vi "HeatFlow Stop Acq Tasks.vi"(9 "HeatFlow HW Cfg":T1, 11 "HeatFlow HW Tasks in":T2) -> (0 "error out":errorcluster)   [LabVIEW 2019, in "Acquisition.lvlib"]
doc: "Perform the acquisition. Replace the contents of this diagram with calls to acquisition hardware."
uses:
  Acquisition.lvlib
  HeatFlow HW Tasks.ctl
  HeatFlow HW Cfg.ctl
  HeatFlow Acq States.ctl
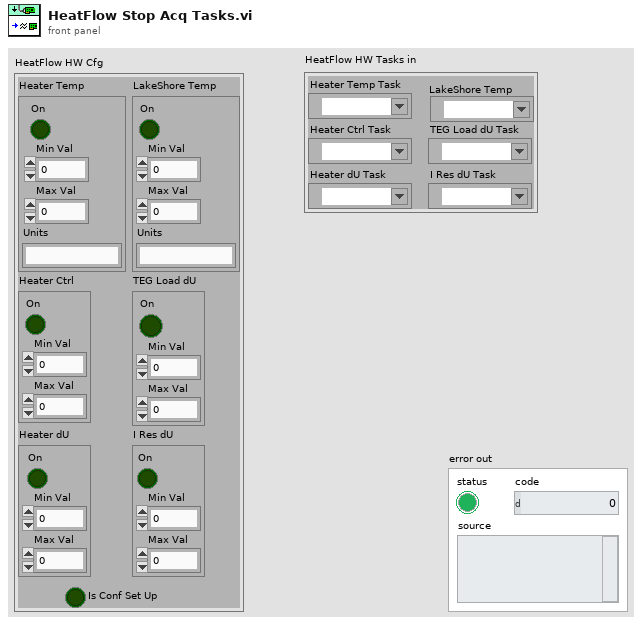
[diagram p1: front panel]
types:
  T1 = typedef "Acquisition.lvlib/HeatFlow HW Cfg.ctl" = cluster{"Heater Temp":cluster{"On":bool, "Min Val":dbl, "Max Val":dbl, "Units":string}, "LakeShore Temp":cluster{"On":bool, "Min Val":dbl, "Max Val":dbl, "Units":string}, "Heater Ctrl":cluster{"On":bool, "Min Val":dbl, "Max Val":dbl}, "TEG Load dU":cluster{"On":bool, "Min Val":dbl, "Max Val":dbl}, "Heater dU":cluster{"On":bool, "Min Val":dbl, "Max Val":dbl}, "I Res dU":cluster{"On":bool, "Min Val":dbl, "Max Val":dbl}, "Is Conf Set Up":bool}
  T2 = typedef "Acquisition.lvlib/HeatFlow HW Tasks.ctl" = cluster{"Heater Temp Task":refnum<k21>, "Heater Ctrl Task":refnum<k21>, "TEG Load dU Task":refnum<k21>, "Heater dU Task":refnum<k21>, "I Res dU Task":refnum<k21>, "LakeShore Temp":refnum<visa-resource-name>}
  T3 = typedef "Acquisition.lvlib/HeatFlow Acq States.ctl" = enum16{"Start", "--- Control ---", "HeaterTemp", "DoControl?", "HeaterCtrl", "--- Readings ---", "DoReadings?", "I_Res_dU", "LakeShoreTemp", "Heater_dU", "TEG_Load_dU", "Calculations", "End"}
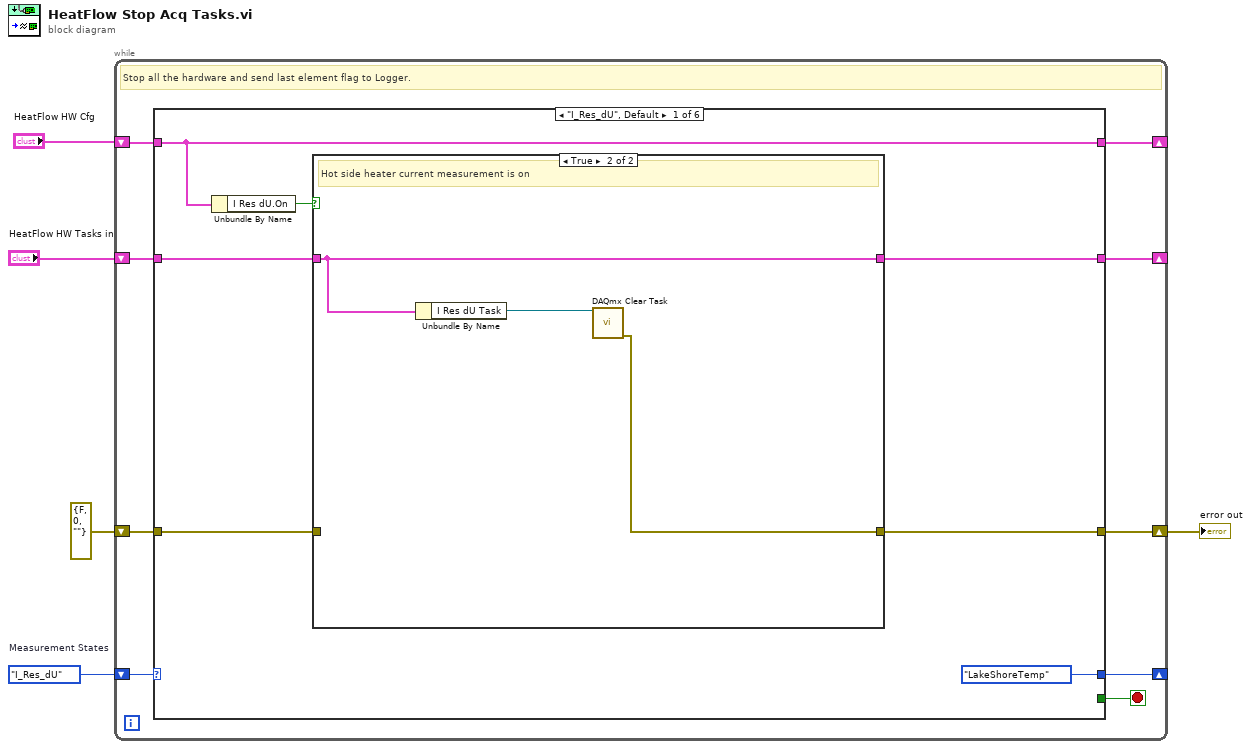
[diagram p0: block diagram]
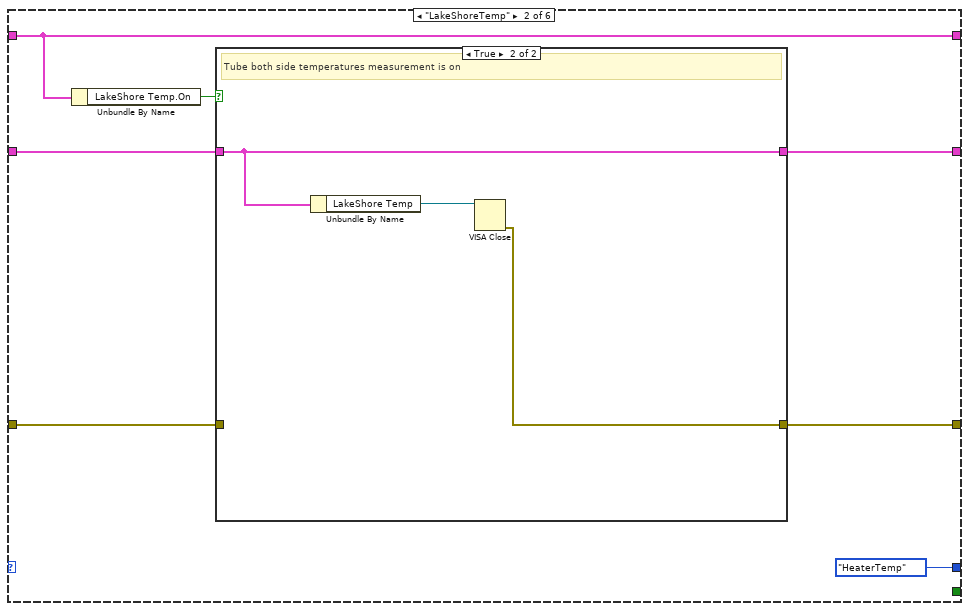
[diagram p3: hidden frame]
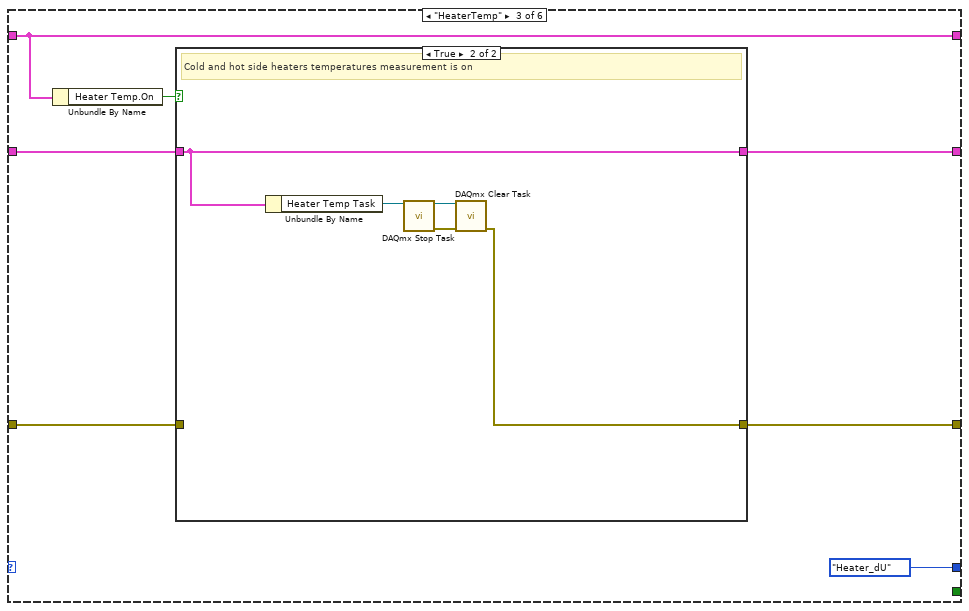
[diagram p5: hidden frame]
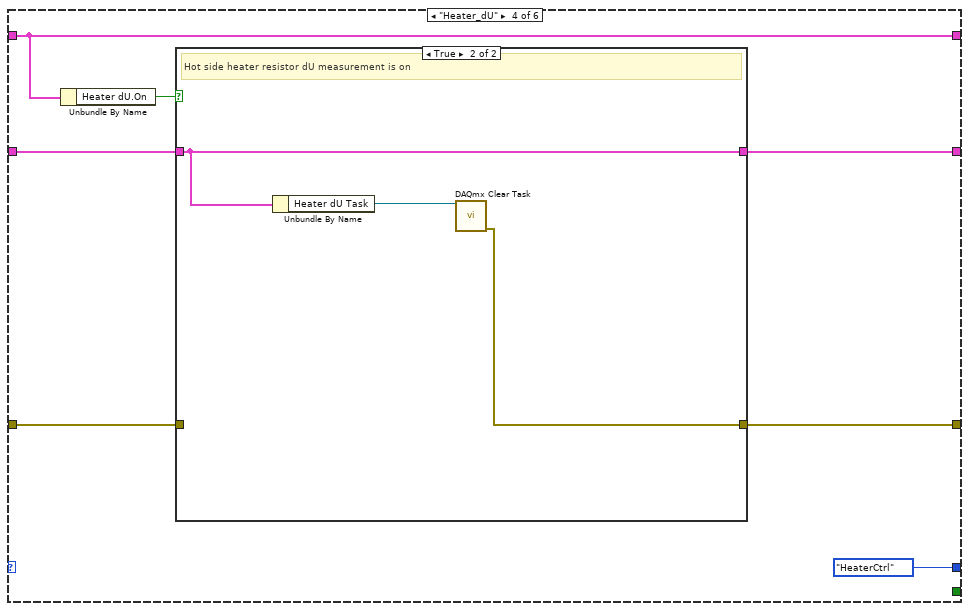
[diagram p7: hidden frame]
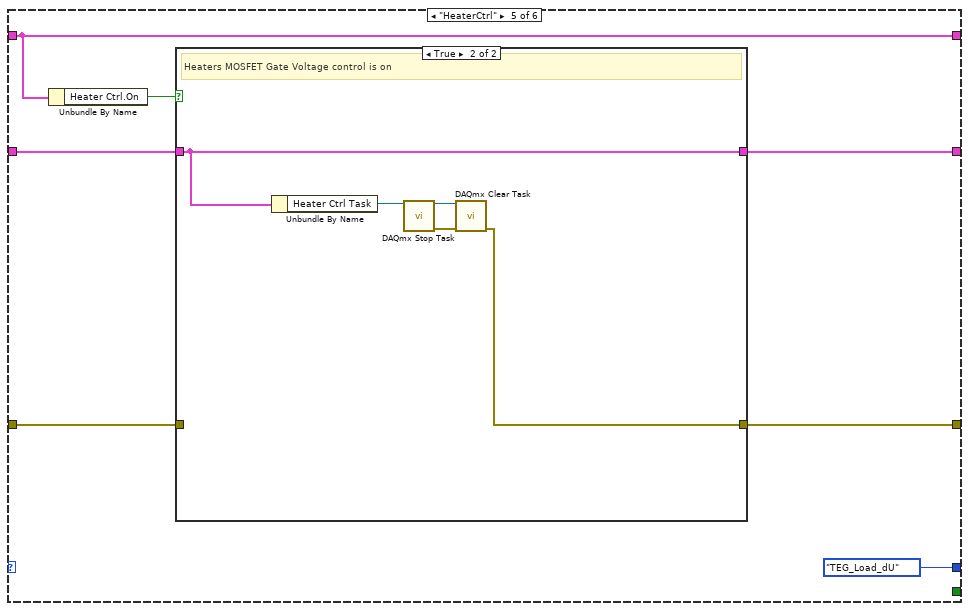
[diagram p9: hidden frame]
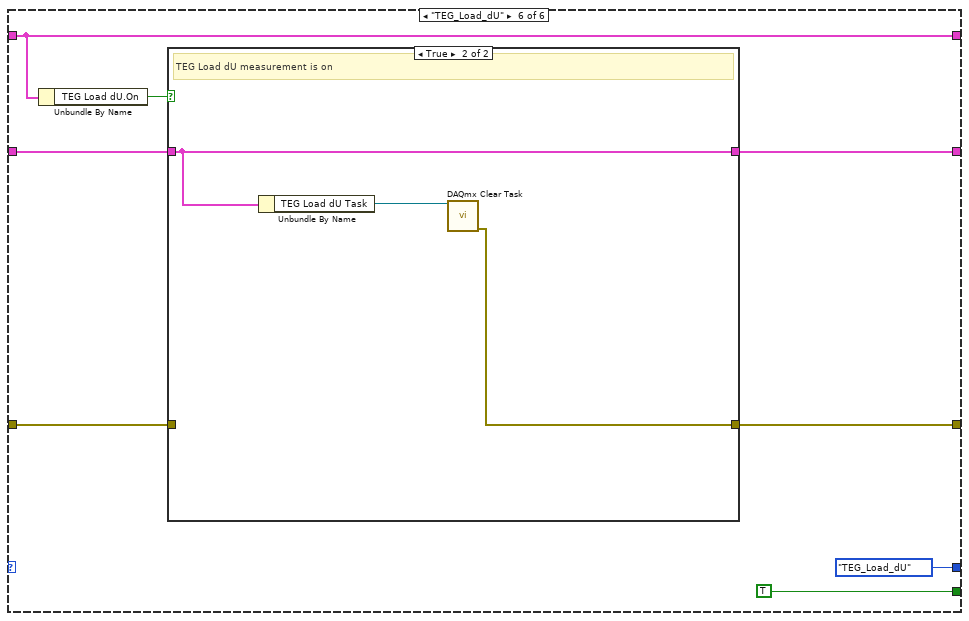
[diagram p11: hidden frame]
diagram:
  w5 = HeatFlow_Acq_States."I_Res_dU"  # Measurement States
  n1 = while {
    shift-right: [w13] -> _
    shift-left: w5 -> [w14]
    shift-right: [w11] -> _
    shift-left: "HeatFlow HW Cfg" -> [w12]
    shift-right: [w7] -> _
    shift-left: "HeatFlow HW Tasks in" -> [w10]
    shift-right: [w8] -> w2
    shift-left: errorcluster {"status"=FALSE, "code"=0, "source"=""} ("error out") -> [w9]
    stop <- w6 stop-if-true
    # "Stop all the hardware and send last element flag to Logger."
    n2 = case shown="\"I_Res_dU\", Default" w14 {
      tunnel: [HeatFlow_Acq_States."LakeShoreTemp" ("Measurement States") HeatFlow_Acq_States."HeaterTemp" ("Measurement States") HeatFlow_Acq_States."Heater_dU" ("Measurement States") HeatFlow_Acq_States."HeaterCtrl" ("Measurement States") HeatFlow_Acq_States."TEG_Load_dU" ("Measurement States") HeatFlow_Acq_States."TEG_Load_dU" ("Measurement States")] -> w13
      tunnel: w12 -> [w20 w32 w44 w58 w70 w85]
      tunnel: [w20 w32 w44 w58 w70 w85] -> w11
      tunnel: [_ _ _ _ _ TRUE] -> w6
      tunnel: w10 -> [w18 w30 w42 w56 w68 w83]
      tunnel: w9 -> [w17 w29 w41 w55 w67 w82]
      tunnel: [w16 w28 w40 w54 w66 w81] -> w8
      tunnel: [w15 w27 w39 w53 w65 w80] -> w7
      frame "I_Res_dU", Default {
        n3 = Unbundle By Name(w20) -> ("I Res dU.On"=w19:bool)
        n4 = case shown="True" w19 {
          tunnel: w18 -> [w23 w26]
          tunnel: w17 -> [w22 _]
          tunnel: [w22 w25] -> w16
          tunnel: [w23 w26] -> w15
          frame False {
            # "Hot side heater current measurement is off"
          }
          frame True {
            # "Hot side heater current measurement is on"
            n5 = Unbundle By Name(w26) -> ("I Res dU Task"=w24:refnum<k21>)
            n6 = call <vilib>:"DAQmx Clear Task.vi"("task in"=w24) -> ("error out"=w25:errorcluster)  [unwired: 14 in]
          }
        }
      }
      frame "LakeShoreTemp" {
        n7 = Unbundle By Name(w32) -> ("LakeShore Temp.On"=w31:bool)
        n8 = case shown="True" w31 {
          tunnel: w30 -> [w35 w38]
          tunnel: w29 -> [w34 _]
          tunnel: [w34 w36] -> w28
          tunnel: [w35 w38] -> w27
          frame False {
            # "Tube both side temperatures measurement is off"
          }
          frame True {
            # "Tube both side temperatures measurement is on"
            n9 = Unbundle By Name(w38) -> ("LakeShore Temp"=w37:refnum<visa-resource-name>)
            n10 = VISA Close(VISA resource name=w37) -> (error out=w36:errorcluster)  [unwired: 1 in]
          }
        }
      }
      frame "HeaterTemp" {
        n11 = Unbundle By Name(w44) -> ("Heater Temp.On"=w43:bool)
        n12 = case shown="True" w43 {
          tunnel: w42 -> [w47 w49]
          tunnel: w41 -> [w46 _]
          tunnel: [w46 w48] -> w40
          tunnel: [w47 w49] -> w39
          frame False {
            # "Cold and hot side heaters temperatures measurement is off"
          }
          frame True {
            # "Cold and hot side heaters temperatures measurement is on"
            n13 = Unbundle By Name(w49) -> ("Heater Temp Task"=w50:refnum<k21>)
            n14 = call <vilib>:"DAQmx Stop Task.vi"("task/channels in"=w50) -> ("task out"=w52:refnum<k21>, "error out"=w51:errorcluster)  [unwired: 13 in]
            n15 = call <vilib>:"DAQmx Clear Task.vi"("task in"=w52, "error in"=w51) -> ("error out"=w48:errorcluster)  [unwired: 13 in]
          }
        }
      }
      frame "Heater_dU" {
        n16 = Unbundle By Name(w58) -> ("Heater dU.On"=w57:bool)
        n17 = case shown="True" w57 {
          tunnel: w56 -> [w61 w64]
          tunnel: w55 -> [w60 _]
          tunnel: [w60 w63] -> w54
          tunnel: [w61 w64] -> w53
          frame False {
            # "Hot side heater resistor dU measurement is off"
          }
          frame True {
            # "Hot side heater resistor dU measurement is on"
            n18 = Unbundle By Name(w64) -> ("Heater dU Task"=w62:refnum<k21>)
            n19 = call <vilib>:"DAQmx Clear Task.vi"("task in"=w62) -> ("error out"=w63:errorcluster)  [unwired: 14 in]
          }
        }
      }
      frame "HeaterCtrl" {
        n20 = Unbundle By Name(w70) -> ("Heater Ctrl.On"=w69:bool)
        n21 = case shown="True" w69 {
          tunnel: w68 -> [w73 w75]
          tunnel: w67 -> [w72 _]
          tunnel: [w72 w74] -> w66
          tunnel: [w73 w75] -> w65
          frame False {
            # "Heaters MOSFET Gate Voltage control is off"
          }
          frame True {
            # "Heaters MOSFET Gate Voltage control is on"
            n22 = Unbundle By Name(w75) -> ("Heater Ctrl Task"=w76:refnum<k21>)
            n23 = call <vilib>:"DAQmx Stop Task.vi"("task/channels in"=w76) -> ("task out"=w78:refnum<k21>, "error out"=w77:errorcluster)  [unwired: 13 in]
            n24 = call <vilib>:"DAQmx Clear Task.vi"("task in"=w78, "error in"=w77) -> ("error out"=w74:errorcluster)  [unwired: 13 in]
          }
        }
      }
      frame "TEG_Load_dU" {
        n25 = Unbundle By Name(w85) -> ("TEG Load dU.On"=w84:bool)
        n26 = case shown="True" w84 {
          tunnel: w83 -> [w88 w91]
          tunnel: w82 -> [w87 _]
          tunnel: [w87 w90] -> w81
          tunnel: [w88 w91] -> w80
          frame False {
            # "TEG Load dU measurement is off"
          }
          frame True {
            # "TEG Load dU measurement is on"
            n27 = Unbundle By Name(w91) -> ("TEG Load dU Task"=w89:refnum<k21>)
            n28 = call <vilib>:"DAQmx Clear Task.vi"("task in"=w89) -> ("error out"=w90:errorcluster)  [unwired: 14 in]
          }
        }
      }
    }
  }
  "error out" <- w2
